vi "StartingBar.vi"() -> ()   [LabVIEW 2014]
doc: "Displays a dialog box complete with a progress bar and cancel button.\n\nThis VI should be called from within a loop with the \"Show\" input set to TRUE, and when the loop exists this VI should be called with \"Show\" set to FALSE."
panel:
  out "Cancel":bool
  in  "Cancel Button":bool
  in  "Show":bool
  out "String":string
  in  "Text":string
  in  "error in (no error)":errorcluster
  out "error out":errorcluster
  in  "Bar Value":dbl
  in  "Max Value (100)":dbl=100.0
  in  "Cancel Button (True)":bool=TRUE
  out "Slide":dbl(slide) scale=0.0..100.0
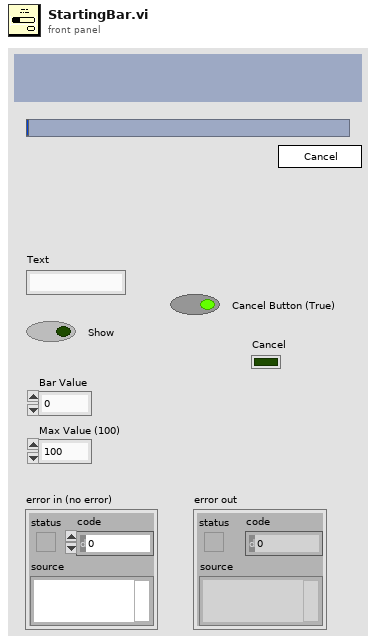
[diagram p1: front panel]
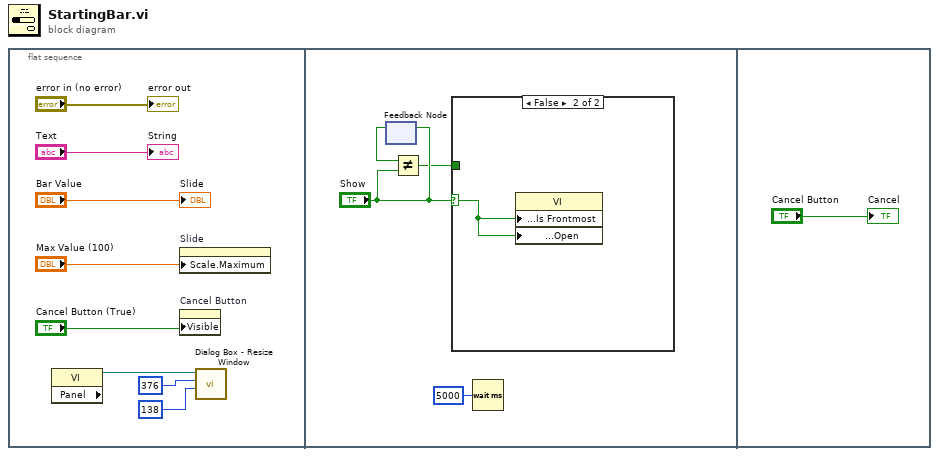
[diagram p0: block diagram]
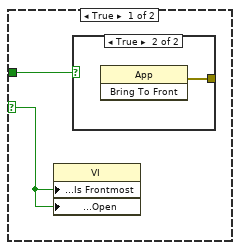
[diagram p2: hidden frame]
diagram:
  n1 = flat-sequence {
    frame #0 {
      n2 = property class="VI" props=["Panel"]() -> (reference out=w3:refnum<vi>)  [unwired: 2 in, 2 out]
      n3 = property on="Slide" class="Slide (strict)"("Scale.Maximum"="Max Value (100)") -> ()  [unwired: 2 in, 2 out]
      n4 = property on="Cancel Button" class="Bool"("Visible"="Cancel Button (True)") -> ()  [unwired: 2 in, 2 out]
      n5 = call "Dialog Box - Resize Window.vi"("Height"=i16 138, "Width"=i16 376, "reference"=w3) -> ()  [unwired: 8 in, 1 out]
      "String" <- "Text"
      "error out" <- "error in (no error)"
      "Slide" <- "Bar Value"
    }
    frame #1 {
      n6 = feedback-in #1("Show") -> ()
      n7 = feedback #1() -> (w11:bool)  [unwired: 1 in]
      n8 = Not Equal?(x=w11, y="Show") -> (x != y?=w10:bool)
      n9 = case shown="False" "Show" {
        selector: "Show" -> [w14 w16]
        tunnel: w10 -> [w13 _]
        frame True {
          n10 = property class="VI"("Front Panel Window:Is Frontmost"=w14, "Front Panel Window:Open"=w14) -> ()  [unwired: 2 in, 2 out]
          n11 = case shown="True" w13 {
            tunnel: [_ w15] -> _
            frame False {
            }
            frame True {
              n12 = invoke class="App" method="Bring To Front"() -> (error out=w15:errorcluster)  [unwired: 3 in, 2 out]
            }
          }
        }
        frame False {
          n13 = property class="VI"("Front Panel Window:Is Frontmost"=w16, "Front Panel Window:Open"=w16) -> ()  [unwired: 2 in, 2 out]
        }
      }
      n14 = Wait (ms)(milliseconds to wait=u32 5000) -> ()  [unwired: 1 out]
    }
    frame #2 {
      "Cancel" <- "Cancel Button"
    }
  }
